vi "drivePower.vi"(10 "speed":dbl, 11 "time":dbl) -> ()   [LabVIEW 2011]
uses:
  drivetrain/gear_shift_state.ctl
  drivetrain/drivetrain_drive_mode.ctl
  drivetrain/drivetrain_drive_write_thread.ctl
  drivetrain/drivetrain_globals.vi
panel:
  out "x+y":u32
  out "unsigned 32bit integer":u32
  out "x > y?":bool
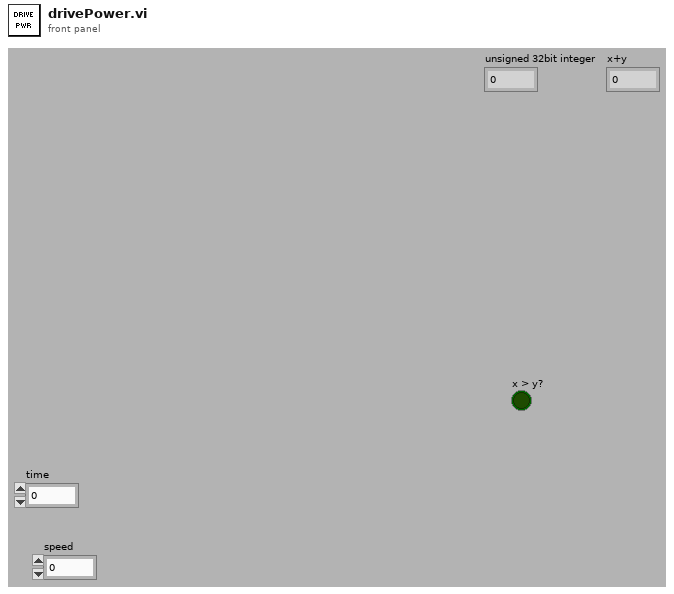
[diagram p1: front panel]
types:
  T1 = typedef "gear_shift_state.ctl" = enum16{"low", "high"}
  T2 = typedef "drivetrain_drive_mode.ctl" = enum16{"open loop", "closed loop"}
  T3 = typedef "drivetrain_drive_write_thread.ctl" = enum16{"Teleop", "Script Engine - Autonomous", "Script Engine - Sequence"}
  T4 = typedef "WPI_RobotDriveDevRef.ctl" = cluster{"DevStatus":errorcluster, "Motors[]":T5[], "Square Inputs":bool, "Max Output":dbl}
  T5 = typedef "WPI_MotorControlDeviceRef.ctl" = cluster{"DeviceStatus":errorcluster, "Type":enum16{"PWM", "CAN"}, "PWM":cluster{"Digital Module":T6, "PWM Channel":T7, "DeadBand":T8}, "CAN":cluster{"Device Number":u8, "Control Mode":T9, "Semaphore":T10, "Max Vout":dbl}, "Invert":bool, "TransformRef":T11, "InvTransformRef":T11}
  T6 = typedef "FPGA_TypedefDigitalModule.ctl" = enum16{"Digital Module 1", "Digital Module 2"}
  T7 = typedef "FPGA_DIOPWMChannel.ctl" = enum8{"PWM 1", "PWM 2", "PWM 3", "PWM 4", "PWM 5", "PWM 6", "PWM 7", "PWM 8", "PWM 9", "PWM 10", "Invalid"}
  T8 = typedef "WPI_PWMDeadband.ctl" = cluster{"Name":string, "maxPositivePwm":i32, "minPositivePwm":i32, "centerPwm":i32, "maxNegativePwm":i32, "minNegativePwm":i32, "angularRange":u16}
  T9 = typedef "WPI_CANJaguar_ControlMode.ctl" = enum8{"Percent VBus", "Current", "Speed", "Position", "Voltage"}
  T10 = typedef "Semaphore RefNum" = refnum<k1>
  T11 = typedef "WPI_PWMTransform_ConPane.ctl" = refnum<vi>
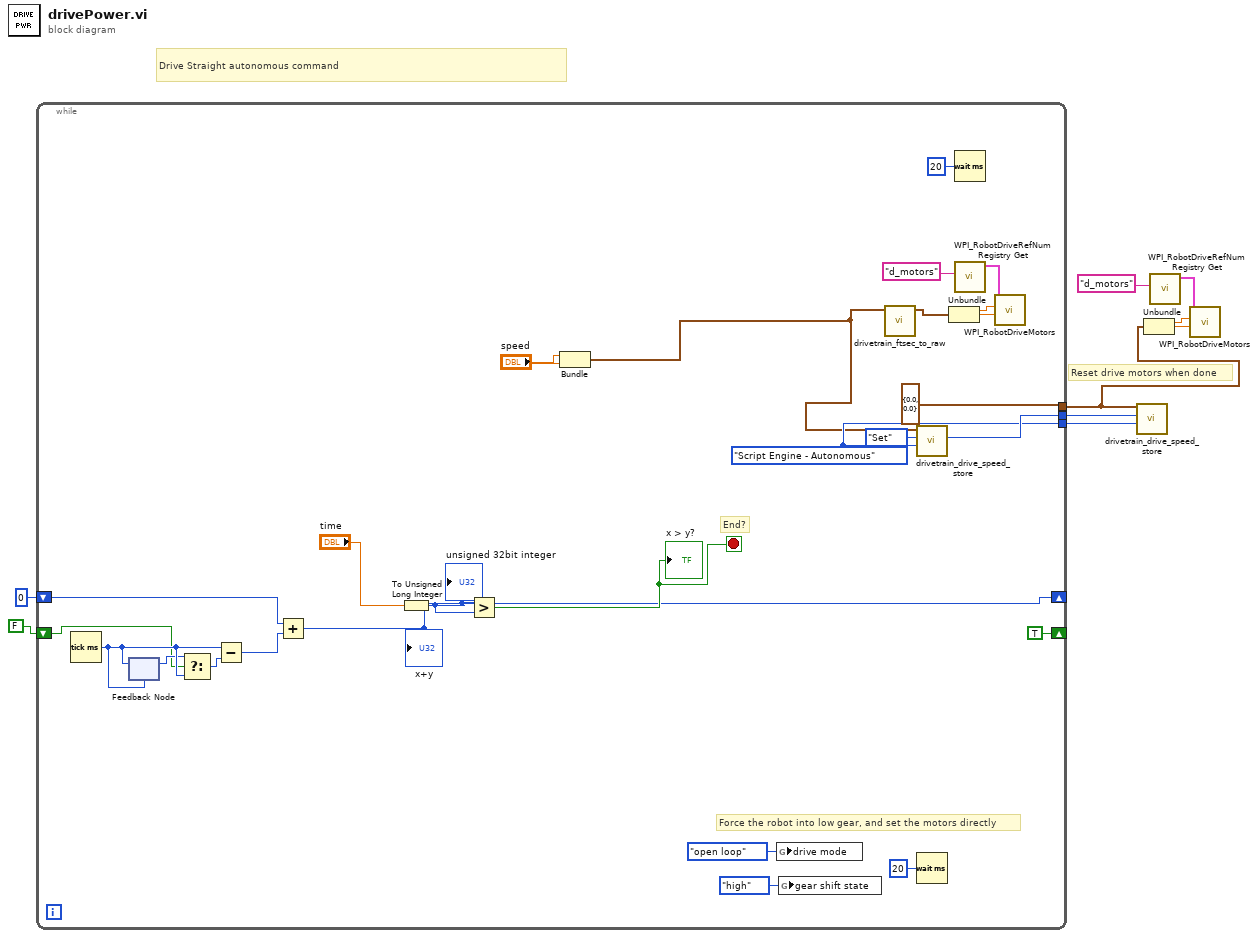
[diagram p0: block diagram]
diagram:
  # "Drive Straight autonomous command"
  # "Reset drive motors when done"
  n1 = while {
    tunnel: [cluster{"Left":dbl, "Right":dbl} {"Left"=0.0, "Right"=0.0} ("Drive")] -> w5
    tunnel: [w32] -> w9
    tunnel: [w31] -> w8
    shift-right: [w20] -> _
    shift-left: u32 0 -> [w23]
    shift-right: [TRUE] -> _
    shift-left: FALSE -> [w13]
    stop <- w21 stop-if-true
    w31 = drivetrain_drive_write_thread."Script Engine - Autonomous" ("Write Thread")
    w32 = enum16{"Set", "Get"}."Set" ("data_store_mode")
    # "End?"
    # "Force the robot into low gear, and set the motors directly"
    n2 = Tick Count (ms)() -> (millisecond timer value=w16:u32)
    n3 = feedback-in #1(w16) -> ()
    n4 = feedback #1(w16) -> (w14:u32)
    n5 = Select(t=w14, s=w13, f=w16) -> (s? t:f=w15:u32)
    n6 = Subtract(x=w16, y=w15) -> (x-y=w22:u32)
    n7 = Add(x=w23, y=w22) -> (x+y=w20:u32)
    "x+y" <- w20
    n8 = To Unsigned Long Integer(number="time") -> (unsigned 32bit integer=w19:u32)
    "unsigned 32bit integer" <- w19
    n9 = Greater?(x=w20, y=w19) -> (0:w21:bool)
    "x > y?" <- w21
    n10 = Bundle("speed"="speed", "speed"="speed") -> (w10:cluster{"speed":dbl, "speed":dbl})  [unwired: 1 in]
    n11 = global write "drivetrain_globals.vi" "drive mode"(drivetrain_drive_mode."open loop" ("drive mode")) -> ()
    n12 = global write "drivetrain_globals.vi" "gear shift state"(gear_shift_state."high" ("gear shift state")) -> ()
    n13 = call "drivetrain_ftsec_to_raw.vi"("Drive Data"=w10) -> ("Drive Data Out"=w24:cluster{"Left":dbl, "Right":dbl})  [unwired: 10 in]
    n14 = call "drivetrain_drive_speed_store.vi"("Write Thread"=w31, "data_store_mode"=w32, "drive data"=w10) -> ()  [unwired: 7 in, 2 out]
    n15 = Wait (ms)(milliseconds to wait=u32 20) -> ()  [unwired: 1 out]
    n16 = Unbundle(w24) -> ("Left"=w26:dbl, "Right"=w27:dbl)
    n17 = Wait (ms)(milliseconds to wait=u32 20) -> ()  [unwired: 1 out]
    n18 = call <vilib>:"WPI_RobotDriveRefNum Registry Get.vi"("refnum name"="d_motors") -> ("RobotDriveDevRef"=w29:T4)  [unwired: 9 in, 1 out]
    n19 = call <vilib>:"WPI_RobotDriveMotors.vi"("RightSpeed"=w27, "LeftSpeed"=w26, "RobotDriveDevRef"=w29) -> ()  [unwired: 7 in, 2 out]
  }
  n20 = call "drivetrain_drive_speed_store.vi"("Write Thread"=w8, "data_store_mode"=w9, "drive data"=w5) -> ()  [unwired: 7 in, 2 out]
  n21 = Unbundle(w5) -> ("Left"=w7:dbl, "Right"=w6:dbl)
  n22 = call <vilib>:"WPI_RobotDriveRefNum Registry Get.vi"("refnum name"="d_motors") -> ("RobotDriveDevRef"=w3:T4)  [unwired: 9 in, 1 out]
  n23 = call <vilib>:"WPI_RobotDriveMotors.vi"("RightSpeed"=w6, "LeftSpeed"=w7, "RobotDriveDevRef"=w3) -> ()  [unwired: 7 in, 2 out]
